vi "contador1_global.vi"() -> ()   [LabVIEW 2017]
panel:
  in  "contador 1":u64
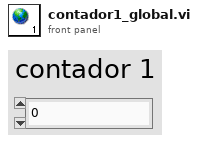
[diagram p1: front panel]
diagram:
